vi "Acknowledge Post Process.vi"(8 "error in (no error)":errorcluster, 9 "Open plot":bool, 10 "Ack Result":refnum<class "Acquired Result.lvclass">, 11 "Monitor-Pulse in":refnum<class "LabActor.lvclass">) -> (0 "error out":errorcluster, 2 "Complete":bool, 3 "Monitor-Pulse out":refnum<class "LabActor.lvclass">)   [LabVIEW 2016, in "LabActor.lvclass"]
uses:
  LabActor.lvclass
  NHMFL_Core/Libraries/Instruments/Results/Acquired Result/Acquired Result.lvclass
  Controllers/Application Controller/Application Controller.lvclass
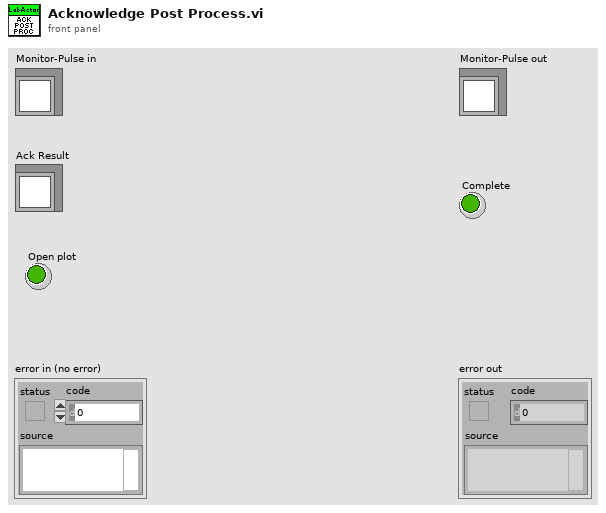
[diagram p1: front panel]
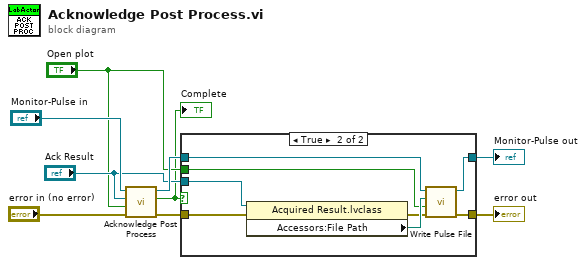
[diagram p0: block diagram]
diagram:
  n1 = call-parent "Acknowledge Post Process.vi"("error in (no error)"="error in (no error)", "Open plot"="Open plot", "Ack Result"="Ack Result", "Monitor-Pulse in"="Monitor-Pulse in") -> ("error out"=w5:errorcluster, "Complete"=w1:bool, "Monitor-Pulse out"=w7:refnum<class "LabActor.lvclass">)  [unwired: 5 in]
  "Complete" <- w1
  n2 = case shown="True" w1 {
    tunnel: w7 -> [w10 w19]
    tunnel: [w10 w18] -> w6
    tunnel: w5 -> [w11 w14]
    tunnel: [w11 w17] -> w4
    tunnel: "Ack Result" -> [_ w16]
    tunnel: "Open plot" -> [_ w12]
    frame False {
    }
    frame True {
      n3 = property class="Acquired Result.lvclass"(reference=w16, error in=w14) -> (error out=w13:errorcluster, "Accessors:File Path"=w15:path)  [unwired: 1 out]
      n4 = call-dynamic "Write Pulse File.vi"("error in (no error)"=w13, "Open plot after pulse"=w12, "Pulse File"=w15, "Monitor-Pulse in"=w19) -> ("error out"=w17:errorcluster, "Monitor-Pulse out"=w18:refnum<class "LabActor.lvclass">)  [unwired: 6 in]
    }
  }
  "error out" <- w4
  "Monitor-Pulse out" <- w6
